vi "RC_COUNT_ALL_DAILY.vi"(0 "Refnum in":T1, 1 "data in":string[][](array[string]), 3 "Array 3":string[](array[string]), 5 "To Date":string, 9 "From Date":string, 11 "error in (no error)":errorcluster, 12 "STATION":i32[](array[numeric]), 14 "SHIFT":i32[](array[numeric])) -> (4 "Refnum out":T1, 6 "data out":string[][](array[string]), 8 "DATE":string[](array[string]), 10 "COUNT":string[](array[string]), 15 "error out":errorcluster)   [LabVIEW 2017]
uses:
  <vilib>/addons/database/Connection.llb/Conn ObjectReference.ctl
  <vilib>/addons/database/NI_Database_API.lvlib
panel:
  in  "Form Date":timestamp
  in  "To Date":timestamp
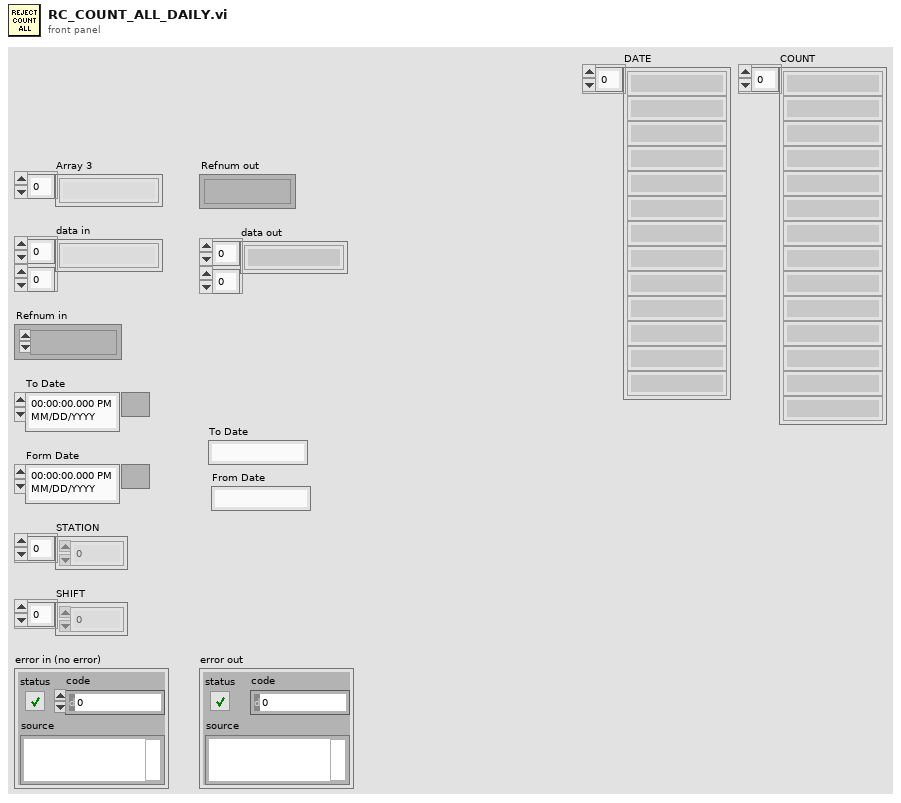
[diagram p1: front panel]
types:
  T1 = typedef "NI_Database_API.lvlib/Conn ObjectReference.ctl" = refnum<k1>
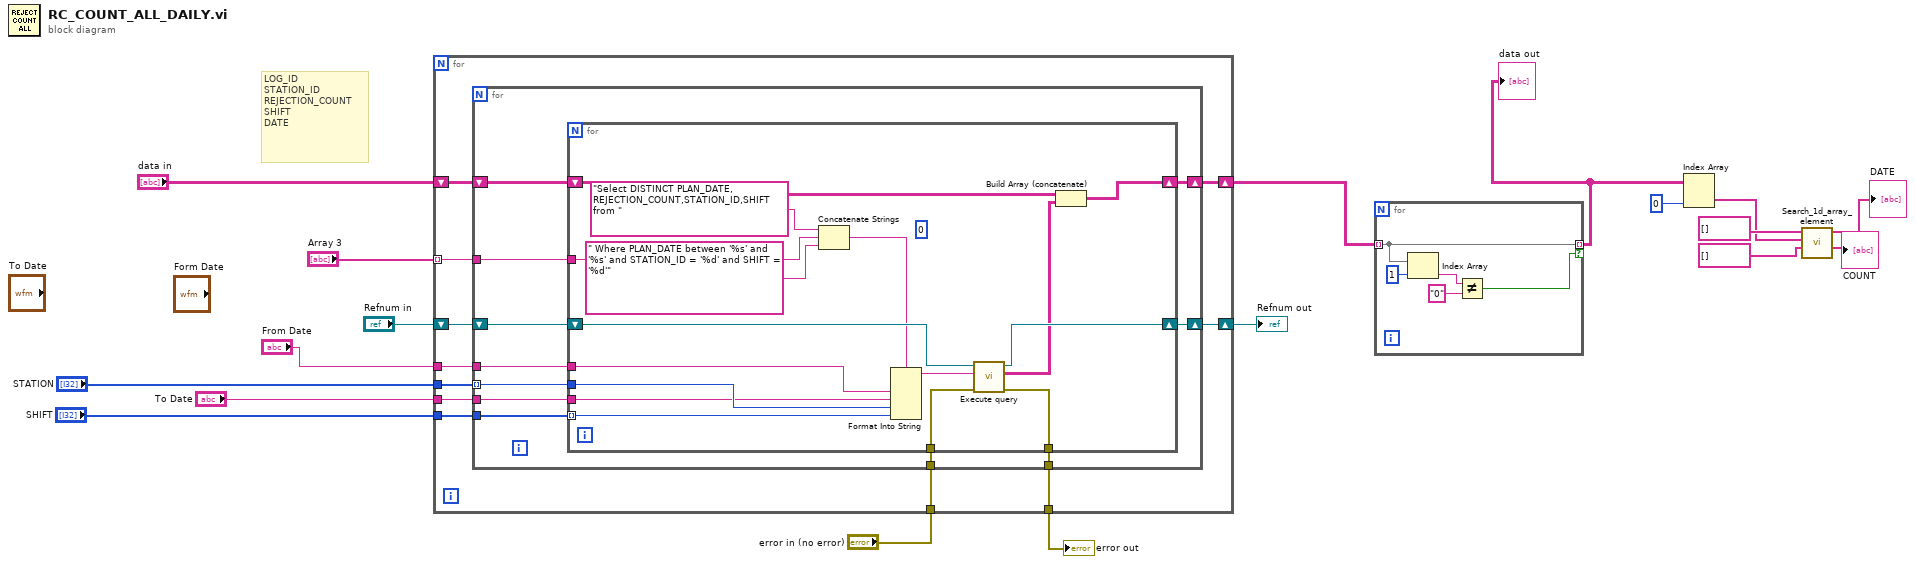
[diagram p0: block diagram]
diagram:
  # "LOG_ID\nSTATION_ID\nREJECTION_COUNT\nSHIFT\nDATE"
  n1 = for {
    tunnel: "To Date" -> [w29]
    tunnel: "From Date" -> [w28]
    shift-right: [w26] -> w11
    shift-left: "Refnum in" -> [w27]
    tunnel: "Array 3" -> [w25] mode=indexing
    shift-right: [w21] -> w4
    shift-left: "data in" -> [w22]
    tunnel: "error in (no error)" -> [w24]
    tunnel: [w23] -> w15
    tunnel: "STATION" -> [w19]
    tunnel: "SHIFT" -> [w20]
    n2 = for {
      tunnel: w29 -> [w40]
      tunnel: w28 -> [w39]
      tunnel: w25 -> [w36]
      tunnel: w20 -> [w31]
      shift-right: [w37] -> w26
      shift-left: w27 -> [w38]
      shift-right: [w32] -> w21
      shift-left: w22 -> [w33]
      tunnel: w19 -> [w30] mode=indexing
      tunnel: w24 -> [w35]
      tunnel: [w34] -> w23
      n3 = for {
        tunnel: w40 -> [w41]
        tunnel: w39 -> [w42]
        tunnel: w36 -> [w54]
        shift-right: [w55] -> w37
        shift-left: w38 -> [w56]
        shift-right: [w50] -> w32
        shift-left: w33 -> [w51]
        tunnel: w31 -> [w43] mode=indexing
        tunnel: w30 -> [w44]
        tunnel: w35 -> [w53]
        tunnel: [w52] -> w34
        (unwired) 0 ("disabled index (col)")
        n4 = Concatenate Strings("Select DISTINCT PLAN_DATE, REJECTION_COUNT,STATION_ID,SHIFT  from ", w54, " Where PLAN_DATE between '%s' and '%s' and STATION_ID = '%d' and SHIFT = '%d'") -> (w47:string)
        n5 = Format Into String(format string=w47, w42, w41, w44, w43) -> (resulting string=w49:string)  [unwired: 2 in, 1 out]
        n6 = call "Execute query.vi"("error in (no error)"=w53, "String"=w49, "connection reference"=w56) -> ("error out"=w52:errorcluster, "Table"=w45:string[][], "connection reference 2"=w55:T1)  [unwired: 3 in, 3 out]
        n7 = Build Array (concatenate)(w51, w45) -> (w50:string[][])
      }
    }
  }
  "error out" <- w15
  "Refnum out" <- w11
  n8 = for {
    tunnel: w4 -> [w58] mode=indexing
    tunnel: [w58] -> w3 mode=indexing if=w57
    n9 = Index Array(array=w58, index=1) -> (element=w60:string)
    n10 = Not Equal?(x=w60, y="0") -> (x != y?=w57:bool)
  }
  "data out" <- w3
  n11 = Index Array(array=w3, index (col)=0 ("disabled index (col)")) -> (element=w8:string[])  [unwired: 1 in]
  n12 = call "Search_1d_array_element.vi"("Count in"=string[] [] ("Count"), "BD Date"=w8, "Elements Found in"=string[] [] ("Elements Found")) -> ("Count out"=→"COUNT":string[], "Elements Found out"=→"DATE":string[])  [unwired: 4 in, 1 out]
